vi "HPGaussianFilter.vi"(2 "Cutoff Radius":dbl min=0.0 max=1.0 format="%.2f", 3 "Image In":T1 {"Dialogs" format="%.0b"}) -> (0 "FFT Out":T1 {"Dialogs" format="%.0b"}, 1 "Image Out":T1 {"Dialogs" format="%.0b"})   [LabVIEW 2024]
doc: "This VI applies a high pass Gaussian filter in the frequency domain. The cutoff ratio is expressed as a percentage of the maximum radius. It only works on greyscale images."
uses:
  <userlib>/ImageProcessing/QTLIB_2595_LV86/QT_Image.ctl
panel:
  # "This VI applies a high pass Gaussian filter in the frequency domain. The cutoff ratio is expressed as a percentage of the maximum radius. It only works on greyscale images."
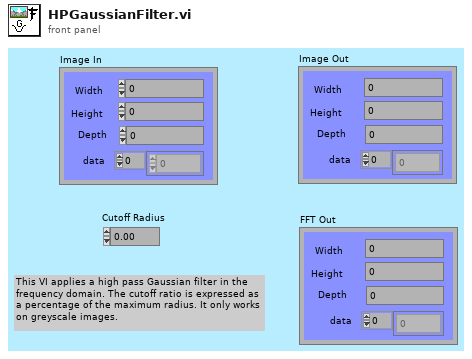
[diagram p1: front panel]
types:
  T1 = typedef "QT_Image.ctl" = cluster{"Width":i32, "Height":i32, "Depth":i32, "data":u8[], "Compressed data":u8[], "Color table":u32[], "Duration":i32, "Options":i32, "Timestamp":i32, "ID":i32, "Reserved":i32, "Dialogs":u32}
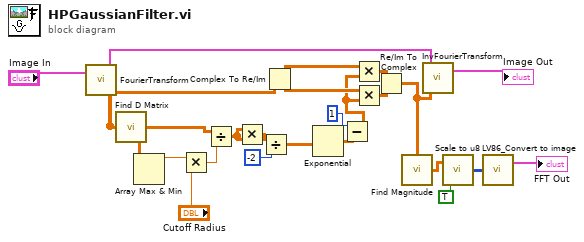
[diagram p0: block diagram]
diagram:
  n1 = call <userlib>:"FourierTransform.vi"("Image In"="Image In") -> ("Complex FT"=w3:cdb[][], "Image Out"=w24:T1)  [unwired: 1 in]
  n2 = call <userlib>:"Find D Matrix.vi"("Complex FT"=w3) -> ("Intensity Graph"=w20:dbl[][])
  n3 = Array Max & Min(array=w20) -> (max value=w10:dbl)  [unwired: 3 out]
  n4 = Multiply(x=w10, y="Cutoff Radius") -> (x*y=w8:dbl)
  n5 = Divide(x=w20, y=w8) -> (x/y=w16:dbl[][])
  n6 = Multiply(x=w16, y=w16) -> (x*y=w15:dbl[][])
  n7 = Divide(x=w15, y=-2 ("x")) -> (x/y=w11:dbl[][])
  n8 = Complex To Re/Im(x + iy=w3) -> (x=w7:dbl[][], y=w6:dbl[][])
  n9 = Exponential(1:w11) -> (0:w14:dbl[][])
  n10 = Subtract(x=1, y=w14) -> (x-y=w2:dbl[][])
  n11 = Multiply(x=w7, y=w2) -> (x*y=w5:dbl[][])
  n12 = Multiply(x=w6, y=w2) -> (x*y=w4:dbl[][])
  n13 = Re/Im To Complex(1:w4, 2:w5) -> (0:w1:cdb[][])
  n14 = call <userlib>:"Find Magnitude.vi"("FFT {X}"=w1) -> ("Magnitude"=w12:dbl[][])
  n15 = call <userlib>:"InvFourierTransform.vi"("Complex matrix"=w1, "Image In"=w24) -> ("Image Out"=→"Image Out":T1)  [unwired: 1 in]
  n16 = call <userlib>:"Scale to u8.vi"("Log scaling?"=TRUE, "Intensity Graph"=w12) -> ("X"=w22:u8[][])
  n17 = call <userlib>:"LV86_Convert to image.vi"("Intensity Graph"=w22) -> ("Image Out"=→"FFT Out":T1)  [unwired: 2 in]
